vi "Execute.vi"(8 "error in (no error)":errorcluster, 11 "Node in":refnum<class "bt_Send_Queue.lvclass">) -> (0 "error out":errorcluster, 1 "Status":T1, 3 "Node out":refnum<class "bt_Send_Queue.lvclass">)   [LabVIEW 2021, in "BT.lvlib" / "bt_Send_Queue.lvclass"]
uses:
  bt_Send_Queue.lvclass
  abs_Node/Status.ctl
  With Values/Send/bt_Send_Synch_WithValues.lvclass/bt_Send_Synch_WithValues.ctl
  bt_Send_Queue.lvclass/bt_Send_Queue.ctl
  With Values/Send/Properties/Read Values.vi
  Properties/Read timeout.vi
  abs_Node/bt_Node.lvclass
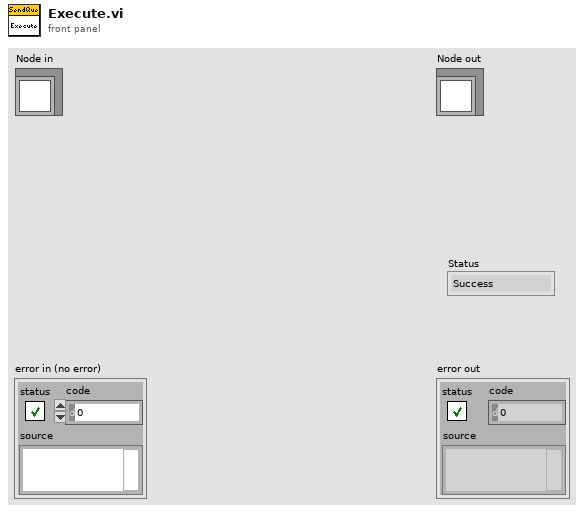
[diagram p1: front panel]
types:
  T1 = typedef "BT.lvlib/bt_Node.lvclass/Status.ctl" = enum16{"Success", "Failure", "Running"}
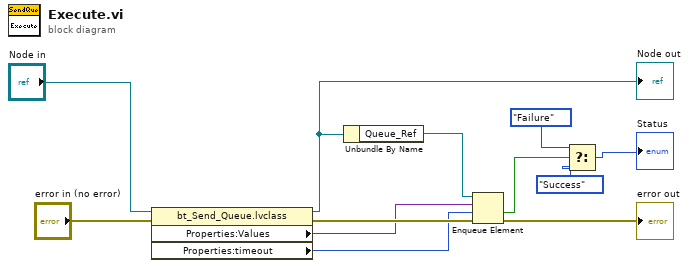
[diagram p0: block diagram]
diagram:
  n1 = property class="bt_Send_Queue.lvclass"(reference="Node in", error in="error in (no error)") -> (reference out=w8:refnum<class "bt_Send_Queue.lvclass">, error out=w11:errorcluster, "Properties:Values"=w7:variant, "Properties:timeout"=w1:i32)
  "Node out" <- w8
  n2 = Unbundle By Name(w8) -> ("Queue_Ref"=w12:refnum<queue>)
  n3 = Enqueue Element(queue=w12, element=w7, timeout in ms (-1)=w1, error in (no error)=w11) -> (timed out?=w5:bool, error out=→"error out":errorcluster)  [unwired: 1 out]
  n4 = Select(t=Status."Failure" ("Status"), s=w5, f=Status."Success" ("Status")) -> (s? t:f=→"Status":T1)
